vi "Resample N Arrays of Pairs (single shot).vi"(0 "Multiple XY-data in":T2(array[cluster]) {"XY-data in"."y" format="%.2p"; "XY-data in"."x" format="%.2p"}, 5 "dt":dbl=1.0 format="%.2p", 7 "t0":dbl=-inf format="%.2p", 9 "interpolation mode":u16(ring)=1 items=["coerce", "linear", "spline", "FIR filter"], 11 "error in (no error)":errorcluster) -> (4 "resampled waveforms out":waveform(dbl)[](array[waveform]), 6 "Multiple XY-data out":T1(array[cluster]) {"XY-data out"."y" format="%.2p"; "XY-data out"."x" format="%.2p"}, 10 "used t0's":dbl[](array[numeric]) format="%.2p", 14 "t0 adjusted warnings":bool[](array[boolean]), 15 "error out":errorcluster)   [LabVIEW 2020, in "NI_MAPro.lvlib"]
doc: "Resamples input waveforms or data according to the user-defined <B>t0</B> and <B>dt</B> values.\n\nWire data to the waveform or data input to determine the polymorphic instance to use or manually select the instance."
uses:
  NI_MAPro.lvlib
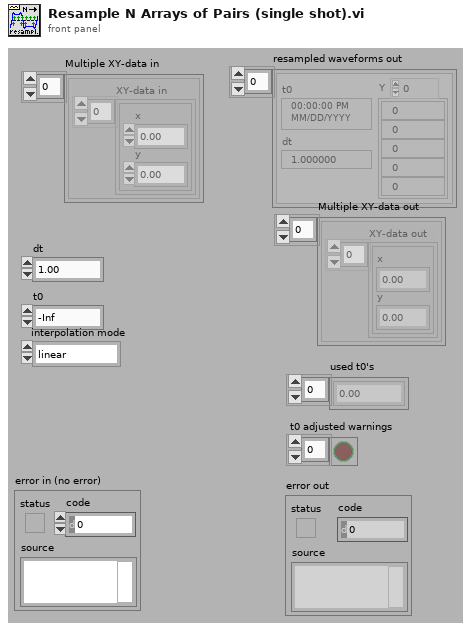
[diagram p1: front panel]
types:
  T1 = cluster{"XY-data out":cluster{"x":dbl, "y":dbl}[]}[]
  T2 = cluster{"XY-data in":cluster{"x":dbl, "y":dbl}[]}[]
  T3 = cluster{"XY-data out":cluster{"x":dbl, "y":dbl}[]}
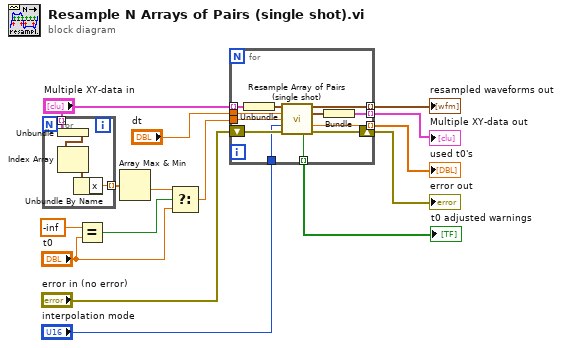
[diagram p0: block diagram]
diagram:
  n1 = for {
    tunnel: "Multiple XY-data in" -> [w19] mode=indexing
    tunnel: [w16] -> w8 mode=indexing
    n2 = Unbundle(w19) -> ("XY-data in"=w18:cluster{"x":dbl, "y":dbl}[])
    n3 = Index Array(array=w18) -> (element=w17:cluster{"x":dbl, "y":dbl})  [unwired: 1 in]
    n4 = Unbundle By Name(w17) -> ("x"=w16:dbl)
  }
  n5 = Equal?(x=-inf, y="t0") -> (x = y?=w3:bool)
  n6 = Array Max & Min(array=w8) -> (min value=w6:dbl)  [unwired: 3 out]
  n7 = Select(t=w6, s=w3, f="t0") -> (s? t:f=w7:dbl)
  n8 = for {
    tunnel: "Multiple XY-data in" -> [w23] mode=indexing
    shift-right: [w30] -> w14
    shift-left: "error in (no error)" -> [w31]
    tunnel: [w29] -> w13 mode=indexing
    tunnel: [w28] -> w12 mode=indexing
    tunnel: [w27] -> w11 mode=indexing
    tunnel: "dt" -> [w26]
    tunnel: w7 -> [w25]
    tunnel: "interpolation mode" -> [w24]
    tunnel: [w20] -> w1 mode=indexing
    n9 = Unbundle(w23) -> ("XY-data in"=w22:cluster{"x":dbl, "y":dbl}[])
    n10 = call "Resample Array of Pairs (single shot).vi"("XY-data in"=w22, "dt"=w26, "t0"=w25, "interpolation mode"=w24, "error in (no error)"=w31) -> ("resampled waveform out"=w28:waveform(dbl), "XY-data out"=w21:cluster{"x":dbl, "y":dbl}[], "used t0"=w29:dbl, "t0 adjusted warning"=w27:bool, "error out"=w30:errorcluster)  [unwired: 6 in]
    n11 = Bundle("XY-data out"=w21) -> (w20:T3)  [unwired: 1 in]
  }
  "error out" <- w14
  "resampled waveforms out" <- w12
  "used t0's" <- w13
  "t0 adjusted warnings" <- w11
  "Multiple XY-data out" <- w1
